vi "PC HOST.vi"() -> ()   [LabVIEW 2020]
panel:
  out "Waveform Graph":dbl[](graph)
  in  "Anode 2":dbl(slide) min=0.0 max=3000.0 scale=0.0..3000.0
  in  "Einzel 2":dbl(slide) min=-10000.0 max=0.0 scale format="%#_6f"
  in  "Initialize":bool
  out "?":string
  in  "Save File Path":path=path "C:/Users/CIBA-Nanolab/Desktop/Implanter-Control-Software/New Text Document.txt"
  in  "Modifier Options":enum32{"Page 1", "Page 2"}(tab)
  in  "PID Anode":bool
  in  "PID Einzel":bool
  in  "stop":bool
  out "?":dbl(graph)
  out "Einzel readback":dbl
  out "readback":dbl
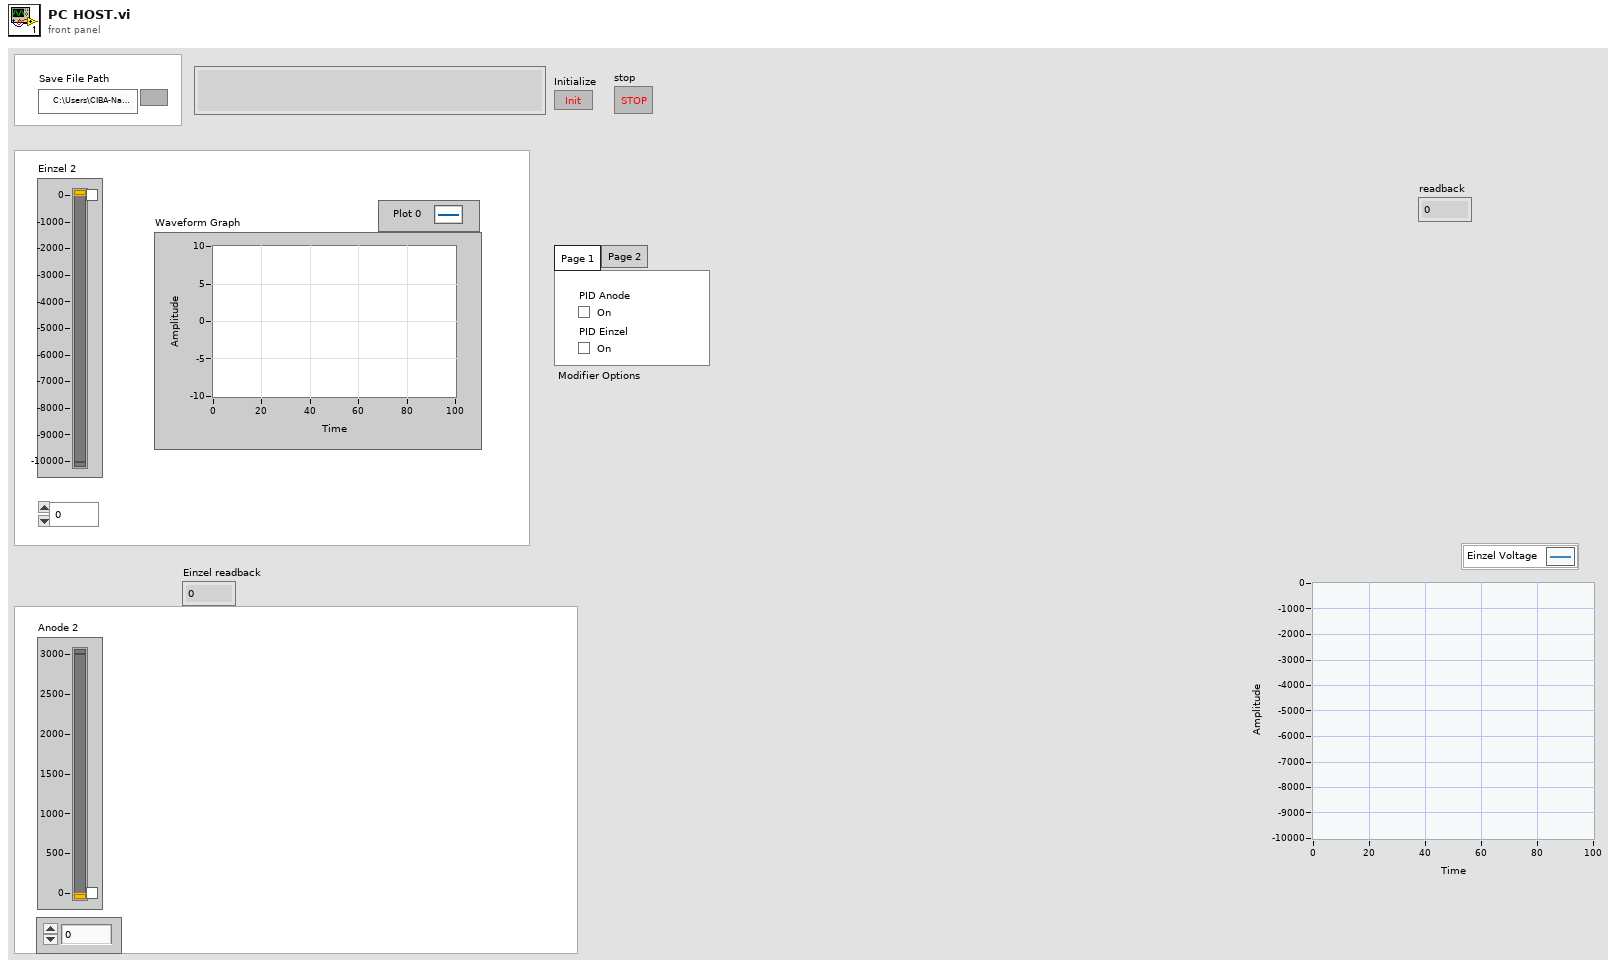
[diagram p1: front panel]
types:
  T1 = enum16{"open", "replace", "create", "open or create", "replace or create", "replace or create with confirmation"}
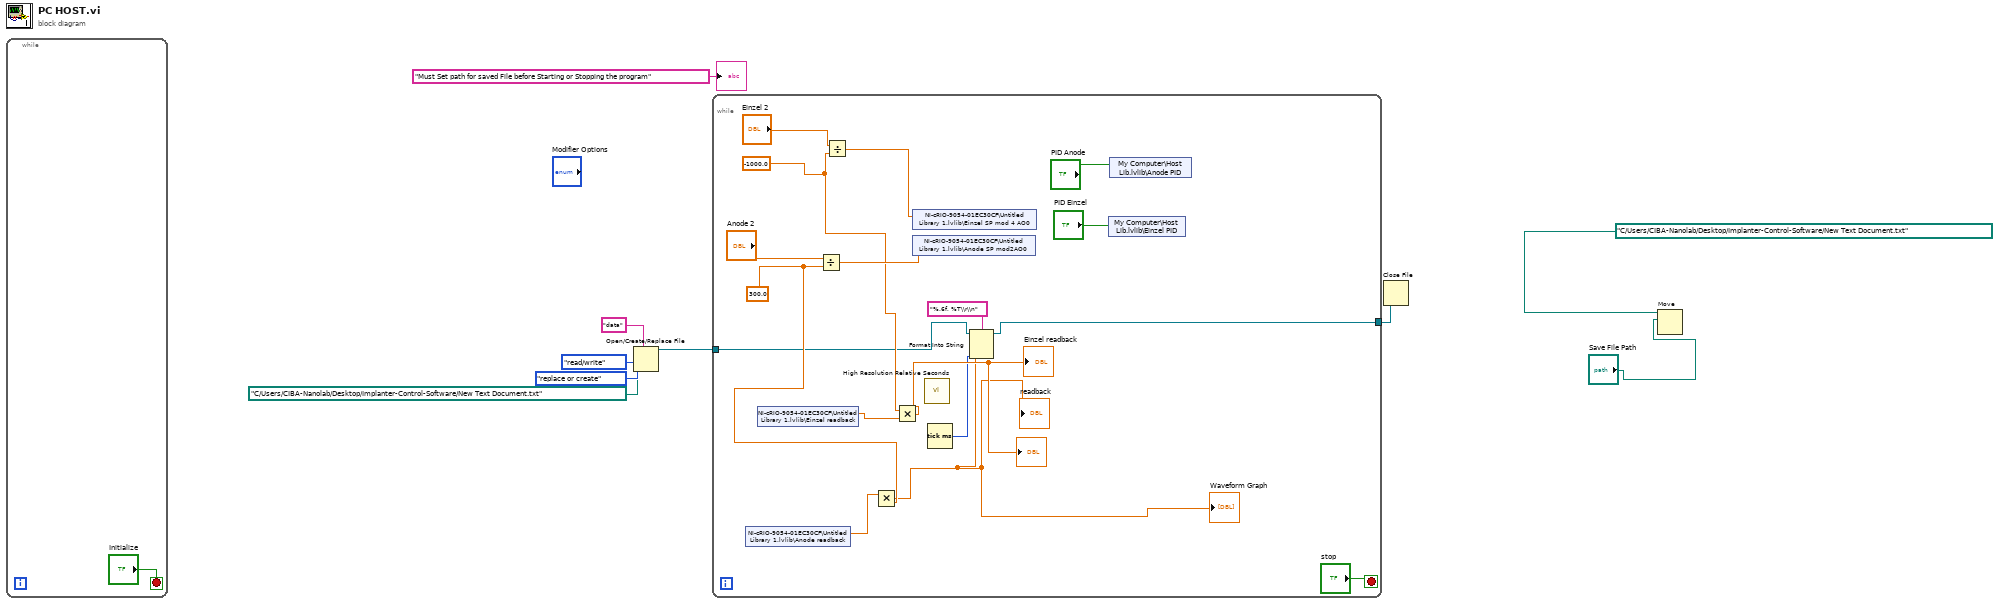
[diagram p0: block diagram]
diagram:
  n1 = while {
    stop <- "Initialize" stop-if-true
  }
  n2 = Open/Create/Replace File(file path (use dialog)=path "C:/Users/CIBA-Nanolab/Desktop/Implanter-Control-Software/New Text Document.txt", prompt="data", operation (0:open)=T1."replace or create", access (0:read/write)=enum16{"read/write", "read-only", "write-only"}."read/write") -> (refnum out=w4:refnum<file>)  [unwired: 2 in, 2 out]
  n3 = while {
    tunnel: [w20] -> w5
    tunnel: w4 -> [w16]
    stop <- "stop" stop-if-true
    w22 = -1000.0
    w24 = 300.0
    n4 = shared-variable "NI-cRIO-9054-01EC30CF\\Untitled Library 1.lvlib\\Anode readback"() -> (w23:dbl)  [unwired: 1 in, 1 out]
    n5 = shared-variable "NI-cRIO-9054-01EC30CF\\Untitled Library 1.lvlib\\Einzel readback"() -> (w21:dbl)  [unwired: 1 in, 1 out]
    n6 = Divide(x="Anode 2", y=w24) -> (x/y=w26:dbl)
    n7 = Divide(x="Einzel 2", y=w22) -> (x/y=w25:dbl)
    n8 = Multiply(x=w23, y=w24) -> (x*y=w11:dbl)
    "readback" <- w11
    "Waveform Graph" <- w11
    n9 = Multiply(x=w22, y=w21) -> (x*y=→"Einzel readback" →"?":dbl)
    n10 = shared-variable "NI-cRIO-9054-01EC30CF\\Untitled Library 1.lvlib\\Einzel SP mod 4 AO0"(w25) -> ()  [unwired: 1 in, 1 out]
    n11 = shared-variable "NI-cRIO-9054-01EC30CF\\Untitled Library 1.lvlib\\Anode SP mod2AO0"(w26) -> ()  [unwired: 1 in, 1 out]
    n12 = call <vilib>:"High Resolution Relative Seconds.vi"() -> ()  [unwired: 1 out]
    n13 = Tick Count (ms)() -> (millisecond timer value=w17:u32)
    n14 = Format Into String(format string="%.6f, %T\\r\\n", initial string=w16, w11, w17) -> (resulting string=w20:refnum<file>)  [unwired: 1 in, 1 out]
    n15 = shared-variable "My Computer\\Host Lib.lvlib\\Einzel PID"("PID Einzel") -> ()  [unwired: 1 in, 1 out]
    n16 = shared-variable "My Computer\\Host Lib.lvlib\\Anode PID"("PID Anode") -> ()  [unwired: 1 in, 1 out]
  }
  n17 = Close File(refnum=w5) -> ()  [unwired: 1 in, 2 out]
  n18 = Move(source path=path "C:/Users/CIBA-Nanolab/Desktop/Implanter-Control-Software/New Text Document.txt", 10:"Save File Path") -> ()  [unwired: 3 in, 3 out]
  "?" <- "Must Set path for saved File before Starting or Stopping the program"
